vi "Init.vi"(3 "Container State":T8={"Indicator?"=TRUE, "Run Mode?"=FALSE, " Refnum"=refnum}, 4 "Previous State":variant, 5 "Previous Version":T7={"Major"=1, "Minor"=0, "Fix"=0, "Build"=0}) -> (2 "Current State":T2={"Graph Visible Items"={"Plot Legend"=TRUE, "Scale Legend"=FALSE, "Graph Palette"=TRUE, "Cursor Legend"=TRUE, "X Scrollbar"=FALSE}, "View Table"=TRUE, "Table Visible Items"={"Vertical Scrollbar"=TRUE, "Horizontal Scrollbar"=TRUE, "Row Headers"=TRUE, "Column Headers"=TRUE, "Vertical Lines"=TRUE, "Horizontal Lines"=TRUE}, "Header Font"={"Font Name"="", "Size"=15, "Bold"=FALSE, "Italic"=FALSE, "Underline"=FALSE, "Strikeout"=FALSE, "Color"=12968}, "Cell Font"={"Font Name"="", "Size"=15, "Bold"=FALSE, "Italic"=FALSE, "Underline"=FALSE, "Strikeout"=FALSE, "Color"=12968}, "Description and Tip..."={"Description"="", "Tip"=""}, "Moveable Splitter Position"=855, "Measurement Cursor Configuration"={"XY"={"enable XY"=FALSE, "Position (X)"=[], "Type"=enum."Absolute", "Y reference"=0.0, "color"=16744512}, "band"={"enable band"=FALSE, "B1"=60.0, "B2"=480.0, "Fixed bandwidth (B2-B1)"=-1.0, "B1 color"=8404992, "B2 color"=8404992}, "harmonic"={"enable harmonics"=FALSE, "X reference (1X)"=100.0, "Maximum"=0, "Subset"=enum."Odd", "1X color"=16744512, "MX color"=16711680}, "sideband"={"enable sideband"=TRUE, "X center (C)"=400.0, "Sidebands"=34, "X spacing (s)"=2.0, "Center color"=16744512, "Sideband color"=16711680}}, "Cursors"={"List"=[], "Tags"=[]}, "X Increment"=1.0, "X Scale"={"Label Visible"=TRUE, "Label Text"="Frequency (Hz)", "Mapping Mode"=0, "Format String"="%.2f"}, "Y Scale"={"Label Visible"=TRUE, "Label Text"="Magnitude", "Mapping Mode"=0, "Format String"="%^_4e"}, "Colors"={"background"=16777215, "major grid"=12632256, "minor grid"=16777215, "font"=12968}, "desired spectrum view"={"scaling"={"linear/dB"=enum."no change", "dB reference"=0.0, "power/magnitude"=enum."no change", "view"=enum."no change"}, "spectral density"=enum."no change"}, "Plot Color Wheel"=[3381759, 32768, 982784, 4375295, 13827953, 13457919, 16757522, 4343295, 16728758, 12095254], "Plots"=[], "registered user events"=variant, "Lock 1X to Peak"=FALSE, "spectrum component"=32, "phase spectrum view"={"desired units"=0, "desired wrapping"=4}} {"phase spectrum view"."desired wrapping" items=["No change", "Unwrap", "Wrap: -360 to 0", "Wrap: -270 to 90", "Wrap: -180 to 180", "Wrap: -90 to 270", "Wrap: 0 to 360", "Wrap: custom range"]; "phase spectrum view"."desired units" items=["No change", "Radians", "Degrees", "Cycles"]; "spectrum component" items=["Magnitude^2"=37, "Magnitude"=32, "Phase"=33, "Real"=34, "Imaginary"=35, "Coherence"=36, "Unknown"=99]; "Y Scale"."Mapping Mode" items=["Linear", "Logarithmic", "dB"]; "X Scale"."Mapping Mode" items=["Linear", "Logarithmic"]})   [LabVIEW 2017, in "Spectrum with Cursors.xctl"]
uses:
  <vilib>/addons/_XControls/Spectrum with Cursors/Spectrum with Cursors.xctl
  <vilib>/addons/_XControls/Spectrum with Cursors/Controls/State.ctl
  <vilib>/Utility/miscctls.llb/LVFontTypeDef.ctl
  <vilib>/addons/_XControls/Spectrum with Cursors/Controls/Measurement Cursor Configuration.ctl
  <vilib>/addons/_NISVFA/_Shared subVIs/Controls/NI Spectrum Component.ctl
  <vilib>/_xctls/Container State.ctl
  <vilib>/_xctls/Version.ctl
  <vilib>/_xctls/XControlSupport.lvlib
panel:
  in  "Tab Control":T1(tab)
  in  "Default Control State":T2={"Graph Visible Items"={"Plot Legend"=FALSE, "Scale Legend"=FALSE, "Graph Palette"=TRUE, "Cursor Legend"=FALSE, "X Scrollbar"=FALSE}, "View Table"=TRUE, "Table Visible Items"={"Vertical Scrollbar"=TRUE, "Horizontal Scrollbar"=TRUE, "Row Headers"=TRUE, "Column Headers"=TRUE, "Vertical Lines"=TRUE, "Horizontal Lines"=TRUE}, "Header Font"={"Font Name"="", "Size"=15, "Bold"=FALSE, "Italic"=FALSE, "Underline"=FALSE, "Strikeout"=FALSE, "Color"=0}, "Cell Font"={"Font Name"="", "Size"=15, "Bold"=FALSE, "Italic"=FALSE, "Underline"=FALSE, "Strikeout"=FALSE, "Color"=0}, "Description and Tip..."={"Description"="", "Tip"=""}, "Moveable Splitter Position"=420, "Measurement Cursor Configuration"={"XY"={"enable XY"=FALSE, "Position (X)"=[], "Type"=enum."Absolute", "Y reference"=0.0, "color"=16744512}, "band"={"enable band"=FALSE, "B1"=60.0, "B2"=480.0, "Fixed bandwidth (B2-B1)"=-1.0, "B1 color"=8404992, "B2 color"=8404992}, "harmonic"={"enable harmonics"=FALSE, "X reference (1X)"=100.0, "Maximum"=10, "Subset"=enum."All", "1X color"=16744512, "MX color"=16711680}, "sideband"={"enable sideband"=FALSE, "X center (C)"=8000.0, "Sidebands"=2, "X spacing (s)"=60.0, "Center color"=16744512, "Sideband color"=16711680}}, "Cursors"={"List"=[], "Tags"=[]}, "X Increment"=1.0, "X Scale"={"Label Visible"=TRUE, "Label Text"="Frequency (Hz)", "Mapping Mode"=0, "Format String"="%.2f"}, "Y Scale"={"Label Visible"=TRUE, "Label Text"="Magnitude", "Mapping Mode"=0, "Format String"="%^_4e"}, "Colors"={"background"=16777215, "major grid"=8355711, "minor grid"=12632256, "font"=0}, "desired spectrum view"={"scaling"={"linear/dB"=enum."no change", "dB reference"=0.0, "power/magnitude"=enum."no change", "view"=enum."no change"}, "spectral density"=enum."no change"}, "Plot Color Wheel"=[3381759, 32768, 982784, 4375295, 13827953, 13457919, 16757522, 4343295, 16728758, 12095254], "Plots"=[], "registered user events"=variant, "Lock 1X to Peak"=FALSE, "spectrum component"=32, "phase spectrum view"={"desired units"=0, "desired wrapping"=4}} {"phase spectrum view"."desired wrapping" items=["No change", "Unwrap", "Wrap: -360 to 0", "Wrap: -270 to 90", "Wrap: -180 to 180", "Wrap: -90 to 270", "Wrap: 0 to 360", "Wrap: custom range"]; "phase spectrum view"."desired units" items=["No change", "Radians", "Degrees", "Cycles"]; "spectrum component" items=["Magnitude^2"=37, "Magnitude"=32, "Phase"=33, "Real"=34, "Imaginary"=35, "Coherence"=36, "Unknown"=99]; "Y Scale"."Mapping Mode" items=["Linear", "Logarithmic", "dB"]; "X Scale"."Mapping Mode" items=["Linear", "Logarithmic"]}
  in  "Default Indicator State":T2={"Graph Visible Items"={"Plot Legend"=FALSE, "Scale Legend"=FALSE, "Graph Palette"=TRUE, "Cursor Legend"=FALSE, "X Scrollbar"=FALSE}, "View Table"=TRUE, "Table Visible Items"={"Vertical Scrollbar"=TRUE, "Horizontal Scrollbar"=TRUE, "Row Headers"=TRUE, "Column Headers"=TRUE, "Vertical Lines"=TRUE, "Horizontal Lines"=TRUE}, "Header Font"={"Font Name"="", "Size"=15, "Bold"=FALSE, "Italic"=FALSE, "Underline"=FALSE, "Strikeout"=FALSE, "Color"=0}, "Cell Font"={"Font Name"="", "Size"=15, "Bold"=FALSE, "Italic"=FALSE, "Underline"=FALSE, "Strikeout"=FALSE, "Color"=0}, "Description and Tip..."={"Description"="", "Tip"=""}, "Moveable Splitter Position"=420, "Measurement Cursor Configuration"={"XY"={"enable XY"=FALSE, "Position (X)"=[], "Type"=enum."Absolute", "Y reference"=0.0, "color"=16744512}, "band"={"enable band"=FALSE, "B1"=60.0, "B2"=480.0, "Fixed bandwidth (B2-B1)"=-1.0, "B1 color"=8404992, "B2 color"=8404992}, "harmonic"={"enable harmonics"=FALSE, "X reference (1X)"=100.0, "Maximum"=10, "Subset"=enum."All", "1X color"=16744512, "MX color"=16711680}, "sideband"={"enable sideband"=FALSE, "X center (C)"=8000.0, "Sidebands"=2, "X spacing (s)"=60.0, "Center color"=16744512, "Sideband color"=16711680}}, "Cursors"={"List"=[], "Tags"=[]}, "X Increment"=1.0, "X Scale"={"Label Visible"=TRUE, "Label Text"="Frequency (Hz)", "Mapping Mode"=0, "Format String"="%.2f"}, "Y Scale"={"Label Visible"=TRUE, "Label Text"="Magnitude", "Mapping Mode"=0, "Format String"="%^_4e"}, "Colors"={"background"=16777215, "major grid"=8355711, "minor grid"=12632256, "font"=0}, "desired spectrum view"={"scaling"={"linear/dB"=enum."no change", "dB reference"=0.0, "power/magnitude"=enum."no change", "view"=enum."no change"}, "spectral density"=enum."no change"}, "Plot Color Wheel"=[3381759, 32768, 982784, 4375295, 13827953, 13457919, 16757522, 4343295, 16728758, 12095254], "Plots"=[], "registered user events"=variant, "Lock 1X to Peak"=FALSE, "spectrum component"=32, "phase spectrum view"={"desired units"=0, "desired wrapping"=4}} {"phase spectrum view"."desired wrapping" items=["No change", "Unwrap", "Wrap: -360 to 0", "Wrap: -270 to 90", "Wrap: -180 to 180", "Wrap: -90 to 270", "Wrap: 0 to 360", "Wrap: custom range"]; "phase spectrum view"."desired units" items=["No change", "Radians", "Degrees", "Cycles"]; "spectrum component" items=["Magnitude^2"=37, "Magnitude"=32, "Phase"=33, "Real"=34, "Imaginary"=35, "Coherence"=36, "Unknown"=99]; "Y Scale"."Mapping Mode" items=["Linear", "Logarithmic", "dB"]; "X Scale"."Mapping Mode" items=["Linear", "Logarithmic"]}
  in  "Default Indicator State 1.0.0.0":T6={"Graph Visible Items"={"Plot Legend"=FALSE, "Scale Legend"=FALSE, "Graph Palette"=TRUE, "Cursor Legend"=FALSE, "X Scrollbar"=FALSE}, "View Table"=TRUE, "Table Visible Items"={"Vertical Scrollbar"=TRUE, "Horizontal Scrollbar"=TRUE, "Row Headers"=TRUE, "Column Headers"=TRUE, "Vertical Lines"=TRUE, "Horizontal Lines"=TRUE}, "Header Font"={"Font Name"="", "Size"=13, "Bold"=FALSE, "Italic"=FALSE, "Underline"=FALSE, "Strikeout"=FALSE, "Color"=0}, "Cell Font"={"Font Name"="", "Size"=13, "Bold"=FALSE, "Italic"=FALSE, "Underline"=FALSE, "Strikeout"=FALSE, "Color"=0}, "Description and Tip..."={"Description"="", "Tip"=""}, "Moveable Splitter Position"=420, "Measurement Cursor Configuration"={"XY"={"enable XY"=FALSE, "Position (X)"=[], "Type"=enum."Absolute", "Y reference"=0.0, "color"=16744512}, "harmonic"={"enable harmonics"=FALSE, "X reference (1X)"=60.0, "Subset"=enum."All", "Maximum"=10, "1X color"=16744512, "MX color"=16711680}, "sideband"={"enable sideband"=FALSE, "X center (C)"=8000.0, "X spacing (s)"=60.0, "Sidebands"=2, "Center color"=16744512, "Sideband color"=16711680}, "integral"={"enable integrating"=FALSE, "X start (L)"=20.0, "X stop (H)"=20000.0, "Fixed bandwidth (H-L)"=-1.0, "color"=16744512}, "differential"={"enable differential"=FALSE, "X1"=1000.0, "X2"=3000.0, "Fixed bandwidth (X2-X1)"=-1.0, "color"=16744512}}, "Cursors"=[], "X Increment"=0.0, "X Scale"={"Label Visible"=TRUE, "Label Text"="Frequency (Hz)", "Mapping Mode"=0, "Format String"="%.2f"}, "Y Scale"={"Label Visible"=TRUE, "Label Text"="Magnitude", "Mapping Mode"=0, "Format String"="%^_4e"}} caption="Default Indicator State (1.0.0.0)" {"Y Scale"."Mapping Mode" items=["Linear", "Logarithmic", "dB"]; "X Scale"."Mapping Mode" items=["Linear", "Logarithmic"]}
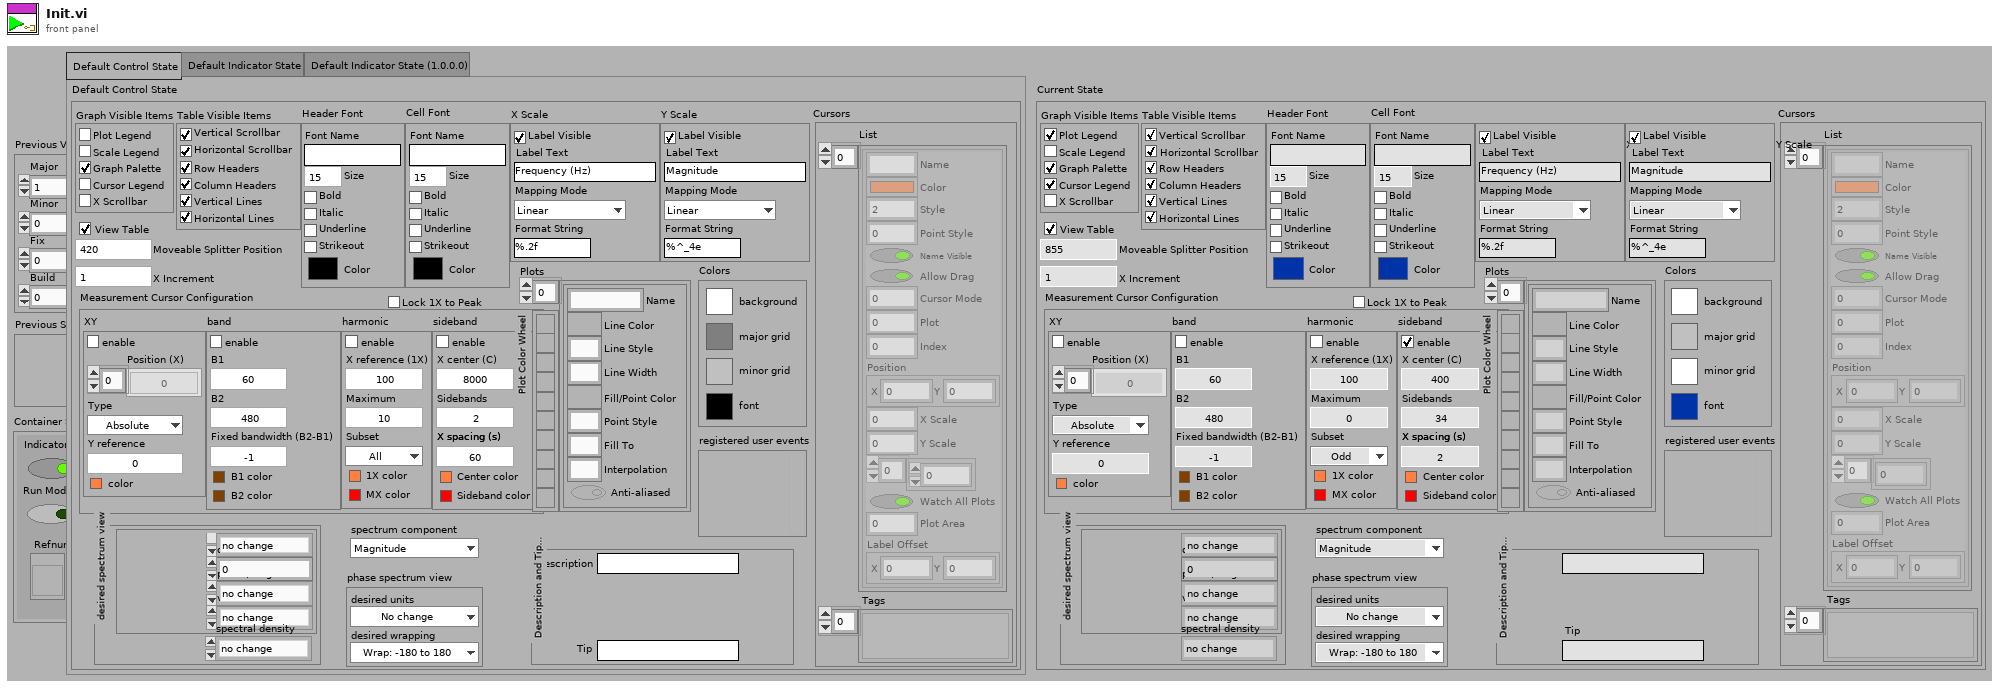
[diagram p1: front panel]
types:
  T1 = enum32{"Default Control State", "Default Indicator State", "Default Indicator State (1.0.0.0)"}
  T2 = typedef "Spectrum with Cursors.xctl/State.ctl" = cluster{"Graph Visible Items":cluster{"Plot Legend":bool, "Scale Legend":bool, "Graph Palette":bool, "Cursor Legend":bool, "X Scrollbar":bool}, "View Table":bool, "Table Visible Items":cluster{"Vertical Scrollbar":bool, "Horizontal Scrollbar":bool, "Row Headers":bool, "Column Headers":bool, "Vertical Lines":bool, "Horizontal Lines":bool}, "Header Font":T3, "Cell Font":T3, "Description and Tip...":cluster{"Description":string, "Tip":string}, "Moveable Splitter Position":i32, "Measurement Cursor Configuration":T4, "Cursors":cluster{"List":cluster{"Name":string, "Color":u32, "Style":i32, "Point Style":u8, "Name Visible":bool, "Allow Drag":bool, "Cursor Mode":u32, "Plot":i32, "Index":i32, "Position":cluster{"X":dbl, "Y":dbl}, "X Scale":u32, "Y Scale":u32, "Watch Plots":i32[], "Watch All Plots":bool, "Plot Area":i32, "Label Offset":cluster{"X":dbl, "Y":dbl}}[], "Tags":variant[]}, "X Increment":dbl, "X Scale":cluster{"Label Visible":bool, "Label Text":string, "Mapping Mode":u8, "Format String":string}, "Y Scale":cluster{"Label Visible":bool, "Label Text":string, "Mapping Mode":u8, "Format String":string}, "Colors":cluster{"background":u32, "major grid":u32, "minor grid":u32, "font":u32}, "desired spectrum view":cluster{"scaling":cluster{"linear/dB":enum16{"no change", "linear", "dB"}, "dB reference":dbl, "power/magnitude":enum16{"no change", "power", "magnitude"}, "view":enum16{"no change", "rms", "peak", "peak-peak"}}, "spectral density":enum16{"no change", "spectrum", "spectral density"}}, "Plot Color Wheel":u32[], "Plots":cluster{"Name":string, "Line Color":u32, "Line Style":u8, "Line Width":u8, "Fill/Point Color":u32, "Point Style":u8, "Fill To":i16, "Interpolation":u8, "Anti-aliased":bool}[], "registered user events":variant, "Lock 1X to Peak":bool, "spectrum component":T5, "phase spectrum view":cluster{"desired units":u16, "desired wrapping":u16}}
  T3 = typedef "LVFontTypeDef.ctl" = cluster{"Font Name":string, "Size":u16, "Bold":bool, "Italic":bool, "Underline":bool, "Strikeout":bool, "Color":u32}
  T4 = typedef "Spectrum with Cursors.xctl/Measurement Cursor Configuration.ctl" = cluster{"XY":cluster{"enable XY":bool, "Position (X)":dbl[], "Type":enum16{"Absolute", "Relative"}, "Y reference":dbl, "color":u32}, "band":cluster{"enable band":bool, "B1":dbl, "B2":dbl, "Fixed bandwidth (B2-B1)":dbl, "B1 color":u32, "B2 color":u32}, "harmonic":cluster{"enable harmonics":bool, "X reference (1X)":dbl, "Maximum":i32, "Subset":enum16{"All", "Even", "Odd"}, "1X color":u32, "MX color":u32}, "sideband":cluster{"enable sideband":bool, "X center (C)":dbl, "Sidebands":i32, "X spacing (s)":dbl, "Center color":u32, "Sideband color":u32}}
  T5 = typedef "NI Spectrum Component.ctl" = u16
  T6 = cluster{"Graph Visible Items":cluster{"Plot Legend":bool, "Scale Legend":bool, "Graph Palette":bool, "Cursor Legend":bool, "X Scrollbar":bool}, "View Table":bool, "Table Visible Items":cluster{"Vertical Scrollbar":bool, "Horizontal Scrollbar":bool, "Row Headers":bool, "Column Headers":bool, "Vertical Lines":bool, "Horizontal Lines":bool}, "Header Font":T3, "Cell Font":T3, "Description and Tip...":cluster{"Description":string, "Tip":string}, "Moveable Splitter Position":i32, "Measurement Cursor Configuration":cluster{"XY":cluster{"enable XY":bool, "Position (X)":dbl[], "Type":enum16{"Absolute", "Relative"}, "Y reference":dbl, "color":u32}, "harmonic":cluster{"enable harmonics":bool, "X reference (1X)":dbl, "Subset":enum16{"All", "Even", "Odd"}, "Maximum":i32, "1X color":u32, "MX color":u32}, "sideband":cluster{"enable sideband":bool, "X center (C)":dbl, "X spacing (s)":dbl, "Sidebands":i32, "Center color":u32, "Sideband color":u32}, "integral":cluster{"enable integrating":bool, "X start (L)":dbl, "X stop (H)":dbl, "Fixed bandwidth (H-L)":dbl, "color":u32}, "differential":cluster{"enable differential":bool, "X1":dbl, "X2":dbl, "Fixed bandwidth (X2-X1)":dbl, "color":u32}}, "Cursors":cluster{"ref":refnum<vi>, "tags":variant}[], "X Increment":dbl, "X Scale":cluster{"Label Visible":bool, "Label Text":string, "Mapping Mode":u8, "Format String":string}, "Y Scale":cluster{"Label Visible":bool, "Label Text":string, "Mapping Mode":u8, "Format String":string}}
  T7 = typedef "XControlSupport.lvlib/Version.ctl" = cluster{"Major":u16, "Minor":u16, "Fix":u16, "Build":u16}
  T8 = typedef "XControlSupport.lvlib/Container State.ctl" = cluster{"Indicator?":bool, "Run Mode?":bool, " Refnum":refnum<vi>}
  T9 = cluster{"desired units":u16, "desired wrapping":u16}
  T10 = cluster{"desired scaling":cluster{"linear/dB":enum16{"no change", "linear", "dB"}, "dB reference (0: no change)":dbl, "power/magnitude":enum16{"no change", "power", "magnitude"}, "view":enum16{"no change", "rms", "peak", "peak-peak"}}, "spectral density desired":enum16{"no change", "spectrum", "spectral density"}}
  T11 = cluster{"background":u32, "major grid":u32, "minor grid":u32, "font":u32}
  T12 = cluster{"Plot Legend":bool, "Scale Legend":bool, "Graph Palette":bool, "Cursor Legend":bool, "X Scrollbar":bool}
  T13 = cluster{"Vertical Scrollbar":bool, "Horizontal Scrollbar":bool, "Row Headers":bool, "Column Headers":bool, "Vertical Lines":bool, "Horizontal Lines":bool}
  T14 = cluster{"Label Visible":bool, "Label Text":string, "Mapping Mode":u8, "Format String":string}
  T15 = cluster{"enable XY":bool, "Position (X)":dbl[], "Type":enum16{"Absolute", "Relative"}, "Y reference":dbl, "color":u32}
  T16 = cluster{"enable harmonics":bool, "X reference (1X)":dbl, "Subset":enum16{"All", "Even", "Odd"}, "Maximum":i32, "1X color":u32, "MX color":u32}
  T17 = cluster{"enable sideband":bool, "X center (C)":dbl, "X spacing (s)":dbl, "Sidebands":i32, "Center color":u32, "Sideband color":u32}
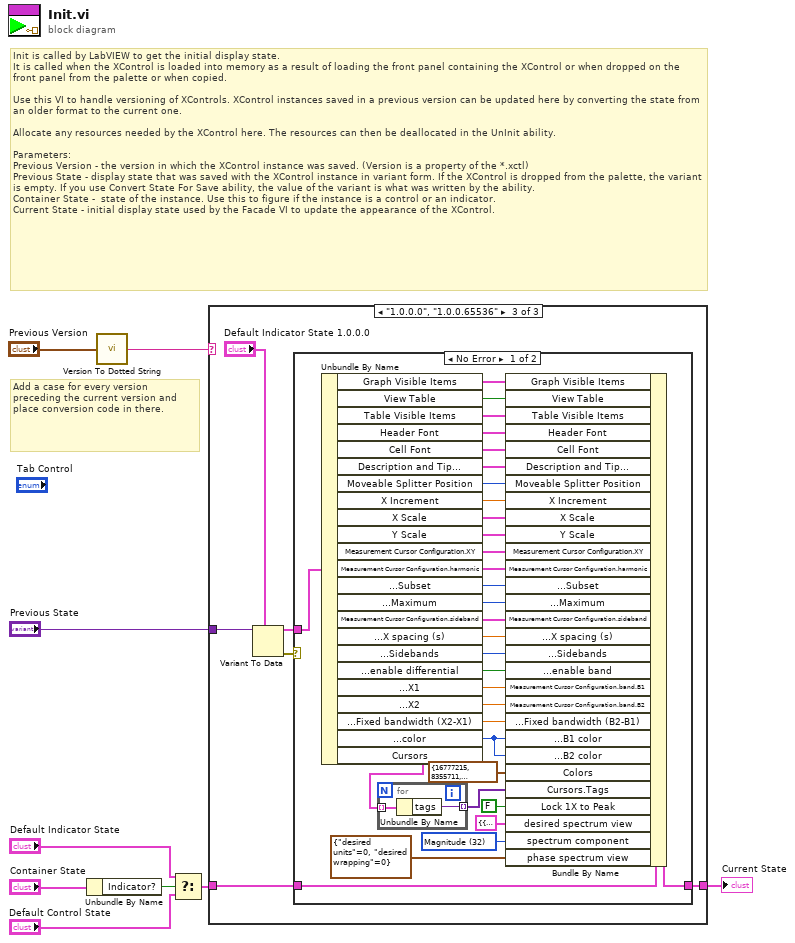
[diagram p0: block diagram]
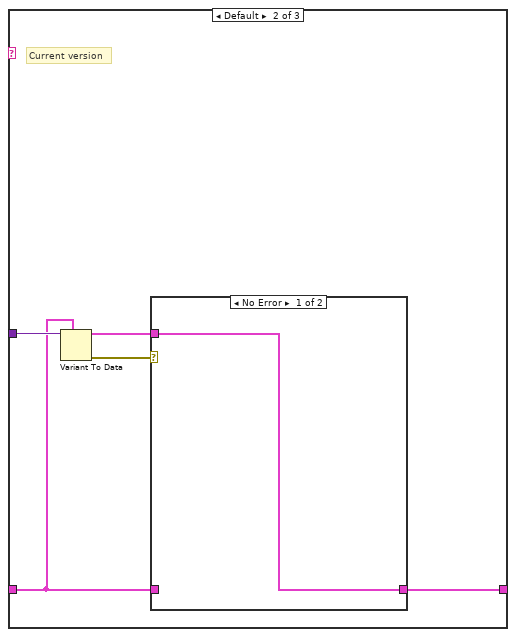
[diagram p3: hidden frame]
diagram:
  # "Add a case for every version preceding the current version and place conversion code in there."
  # "Init is called by LabVIEW to get the initial display state.\nIt is called when the XControl is loaded into memory as a result of loading the front panel containing the XControl or when dropped on the front panel from the palette or when copied.\n\nUse this VI to handle versioning of XControls. XControl instances saved in a previous version can be updated here by converting the state from an older format to the current one.\n\nAllocate any resources needed by the XControl here. The resources can then be deallocated in the UnInit ability.\n\nParameters:\nPrevious Version - the version in which the XControl instance was saved. (Version is a property of the *.xctl)\nPrevious State - display state that was saved with the XControl instance in variant form. If the XControl is dropped from the palette, the variant is empty. If you use Convert State For Save ability, the value of the variant is what was written by the ability. \nContainer State -  state of the instance. Use this to figure if the instance is a control or an indicator.\nCurrent State - initial display state used by the Facade VI to update the appearance of the XControl."
  n1 = Unbundle By Name("Container State") -> ("Indicator?"=w4:bool)
  n2 = call <vilib>:"Version To Dotted String.vi"("Version"="Previous Version") -> ("String Version"=w1:string)
  n3 = Select(t="Default Indicator State", s=w4, f="Default Control State") -> (s? t:f=w3:T2)
  n4 = case shown="\"1.0.0.0\", \"1.0.0.65536\"" w1 {
    tunnel: "Previous State" -> [_ w15 w23]
    tunnel: [w10 w12 w21] -> w8
    tunnel: w3 -> [w10 w11 w19]
    frame "0.0.0.0" {
      # "Just created, use default state"
    }
    frame Default {
      # "Current version"
      n5 = Variant To Data(type=w11, Variant=w15) -> (data=w13:T2, error out=w14:errorcluster)  [unwired: 1 in]
      n6 = case shown="No Error" w14 {
        tunnel: w13 -> [w16 _]
        tunnel: [w16 w17] -> w12
        tunnel: w11 -> [_ w17]
        frame No Error {
        }
        frame Error {
          # "Error converting previously \nsaved state. Use default instead."
        }
      }
    }
    frame "1.0.0.0", "1.0.0.65536" {
      n7 = Variant To Data(type="Default Indicator State 1.0.0.0", Variant=w23) -> (data=w20:T6, error out=w22:errorcluster)  [unwired: 1 in]
      n8 = case shown="No Error" w22 {
        tunnel: w20 -> [w45 _]
        tunnel: [w44 w58] -> w21
        tunnel: w19 -> [w30 w58]
        frame No Error {
          w25 = T5 32 items=["Magnitude^2"=37, "Magnitude"=32, "Phase"=33, "Real"=34, "Imaginary"=35, "Coherence"=36, "Unknown"=99] ("spectrum component")
          n9 = Unbundle By Name(w45) -> ("Graph Visible Items"=w46:T12, "View Table"=w47:bool, "Table Visible Items"=w48:T13, "Header Font"=w49:T3, "Cell Font"=w50:T3, "Description and Tip..."=w51:cluster{"Description":string, "Tip":string}, "Moveable Splitter Position"=w52:i32, "X Increment"=w53:dbl, "X Scale"=w54:T14, "Y Scale"=w55:T14, "Measurement Cursor Configuration.XY"=w42:T15, "Measurement Cursor Configuration.harmonic"=w41:T16, "Measurement Cursor Configuration.harmonic.Subset"=w34:enum16{"All", "Even", "Odd"}, "Measurement Cursor Configuration.harmonic.Maximum"=w33:i32, "Measurement Cursor Configuration.sideband"=w40:T17, "Measurement Cursor Configuration.sideband.X spacing (s)"=w32:dbl, "Measurement Cursor Configuration.sideband.Sidebands"=w31:i32, "Measurement Cursor Configuration.differential.enable differential"=w39:bool, "Measurement Cursor Configuration.differential.X1"=w38:dbl, "Measurement Cursor Configuration.differential.X2"=w37:dbl, "Measurement Cursor Configuration.differential.Fixed bandwidth (X2-X1)"=w36:dbl, "Measurement Cursor Configuration.differential.color"=w35:u32, "Cursors"=w29:cluster{"ref":refnum<vi>, "tags":variant}[])
          n10 = for {
            tunnel: w29 -> [w57] mode=indexing
            tunnel: [w56] -> w28 mode=indexing
            n11 = Unbundle By Name(w57) -> ("tags"=w56:variant)
          }
          n12 = Bundle By Name(cluster=w30, "Graph Visible Items"=w46, "View Table"=w47, "Table Visible Items"=w48, "Header Font"=w49, "Cell Font"=w50, "Description and Tip..."=w51, "Moveable Splitter Position"=w52, "X Increment"=w53, "X Scale"=w54, "Y Scale"=w55, "Measurement Cursor Configuration.XY"=w42, "Measurement Cursor Configuration.harmonic"=w41, "Measurement Cursor Configuration.harmonic.Subset"=w34, "Measurement Cursor Configuration.harmonic.Maximum"=w33, "Measurement Cursor Configuration.sideband"=w40, "Measurement Cursor Configuration.sideband.X spacing (s)"=w32, "Measurement Cursor Configuration.sideband.Sidebands"=w31, "Measurement Cursor Configuration.band.enable band"=w39, "Measurement Cursor Configuration.band.B1"=w38, "Measurement Cursor Configuration.band.B2"=w37, "Measurement Cursor Configuration.band.Fixed bandwidth (B2-B1)"=w36, "Measurement Cursor Configuration.band.B1 color"=w35, "Measurement Cursor Configuration.band.B2 color"=w35, "Colors"=T11 {"background"=16777215, "major grid"=8355711, "minor grid"=12632256, "font"=0}, "Cursors.Tags"=w28, "Lock 1X to Peak"=FALSE, "desired spectrum view"=T10 {"desired scaling"={"linear/dB"=enum."no change", "dB reference (0: no change)"=0.0, "power/magnitude"=enum."no change", "view"=enum."no change"}, "spectral density desired"=enum."no change"} ("spectrum view"), "spectrum component"=w25, "phase spectrum view"=T9 {"desired units"=0, "desired wrapping"=0}) -> (w44:T2)
        }
        frame Error {
          # "Error converting previously \nsaved state. Use default instead."
        }
      }
    }
  }
  "Current State" <- w8
